vi "SPI Engine.Get SPI Transaction Data.vi"(8 "Get New Data":bool, 11 "DLU To SPI Engine Data FIFO":refnum<k21>) -> (0 "Output Valid":bool, 3 "SPI Transaction Data":T1)   [LabVIEW 2013]
uses:
  <vilib>/rvi/DataTransferAndStorage/Container/XNode/niFpgaContainer.xnode
  <vilib>/rvi/FIFO/Fifo_Resource/niFpgaFifoEmulationRefIn.vi
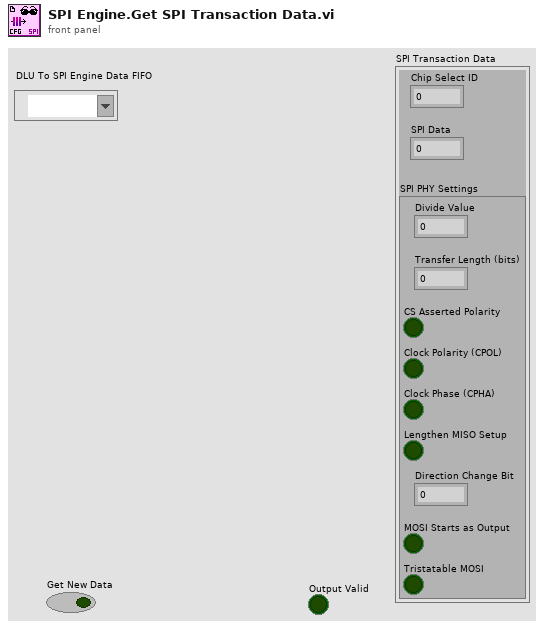
[diagram p1: front panel]
types:
  T1 = cluster{"Chip Select ID":u8, "SPI Data":u64, "SPI PHY Settings":cluster{"Divide Value":u8, "Transfer Length (bits)":u8, "CS Asserted Polarity":bool, "Clock Polarity (CPOL)":bool, "Clock Phase (CPHA)":bool, "Lengthen MISO Setup":bool, "Direction Change Bit":u8, "MOSI Starts as Output":bool, "Tristatable MOSI":bool}}
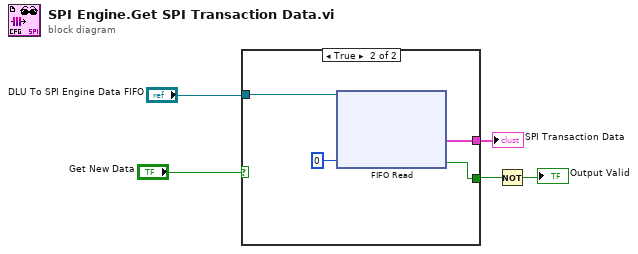
[diagram p0: block diagram]
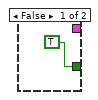
[diagram p2: hidden frame]
diagram:
  n1 = case shown="True" "Get New Data" {
    tunnel: "DLU To SPI Engine Data FIFO" -> [_ w10]
    tunnel: [_ w8] -> w1
    tunnel: [TRUE ("Timed Out?") w7] -> w5
    frame False {
    }
    frame True {
      n2 = xnode "FIFO Read"("Timeout"=0, "FIFO In"=w10) -> ("Element"=w8:T1, "Timed Out?"=w7:bool)  [unwired: 1 out]
    }
  }
  "SPI Transaction Data" <- w1
  n3 = Not(x=w5) -> (.not. x?=→"Output Valid":bool)
